vi "Nigel Tamagotchi Full Actor Launcher.vi"   [LabVIEW 2026]
uses:
  Tamagotchi Full Actor Folder/Tamagotchi Full Actor.lvclass
  <vilib>/ActorFramework/Actor/Actor.lvclass
panel:
  # "Nigel-gotchi loading..."
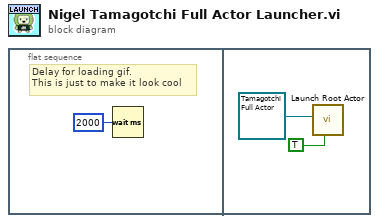
[diagram p0: block diagram]
diagram:
  n1 = flat-sequence {
    frame #0 {
      # "Delay for loading gif.\nThis is just to make it look cool"
      n2 = Wait (ms)(milliseconds to wait=u32 2000) -> ()  [unwired: 1 out]
    }
    frame #1 {
      n3 = call <vilib>:"Launch Root Actor.vi"("Open Actor Core front panel? (F)"=TRUE, "Actor"=refnum<class "Tamagotchi Full Actor.lvclass"> refnum ("Tamagotchi Full Actor.lvclass")) -> ()  [unwired: 8 in, 2 out]
    }
  }
